vi "ferro fit.vi"(7 "ferro response parameters":T1 {"time const b (uS)" scale=0.0..200.0; "amplitude b (V)" scale=0.0..50.0; "time const a (uS)" scale=0.0..200.0; "amplitude a (V)" scale=0.0..50.0}, 11 "time array in (uS)":dbl[](array[numeric])) -> (0 "parameters array out":dbl[](array[numeric]), 2 "voltage array out (V)":dbl[](array[numeric]), 3 "time array out (uS)":dbl[](array[numeric]))   [LabVIEW 2017]
uses:
  typedefs/ferro response parameter cluster.ctl
panel:
  # "needs work\nsee BD"
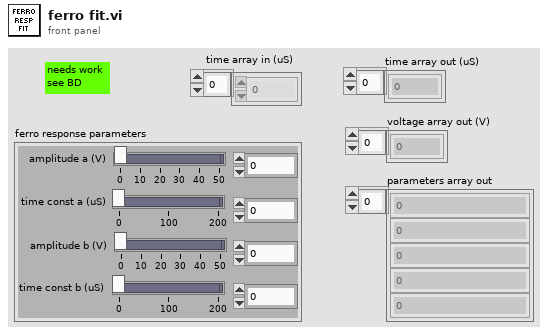
[diagram p1: front panel]
types:
  T1 = typedef "ferro response parameter cluster.ctl" = cluster{"amplitude a (V)":dbl, "time const a (uS)":dbl, "amplitude b (V)":dbl, "time const b (uS)":dbl}
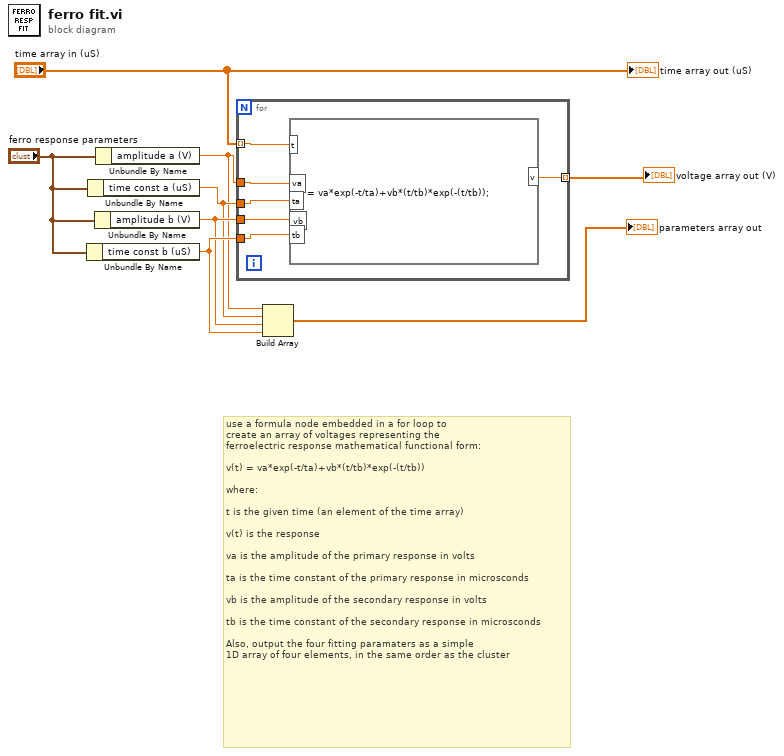
[diagram p0: block diagram]
diagram:
  # "use a formula node embedded in a for loop to \ncreate an array of voltages representing the \nferroelectric response mathematical functional form:\n\nv(t) = va*exp(-t/ta)+vb*(t/tb)*exp(-(t/tb))\n\nwhere:\n\nt is the given time (an element of the time array)\n\nv(t) is the response\n\nva is the amplitude of the primary response in volts\n\nta is the time constant of the primary response in microsconds\n\nvb is the amplitude of the secondary response in volts\n\ntb is the time constant of the secondary response in microsconds\n\nAlso, output the four fitting paramaters as a simple \n1D array of four elements, in the same order as the cluster"
  n1 = Unbundle By Name("ferro response parameters") -> ("time const b (uS)"=w6:dbl)
  n2 = Unbundle By Name("ferro response parameters") -> ("time const a (uS)"=w4:dbl)
  n3 = Unbundle By Name("ferro response parameters") -> ("amplitude b (V)"=w5:dbl)
  n4 = Unbundle By Name("ferro response parameters") -> ("amplitude a (V)"=w3:dbl)
  n5 = for {
    tunnel: w6 -> [w14]
    tunnel: w5 -> [w13]
    tunnel: w4 -> [w12]
    tunnel: w3 -> [w11]
    tunnel: "time array in (uS)" -> [w10] mode=indexing
    tunnel: [w9] -> w1 mode=indexing
    n6 = formula code="v = va*exp(-t/ta)+vb*(t/tb)*exp(-(t/tb));"("va"=w11, "ta"=w12, "vb"=w13, "tb"=w14, "t"=w10) -> ("v"=w9:dbl)
  }
  "voltage array out (V)" <- w1
  n7 = Build Array(w3, w4, w5, w6) -> (→"parameters array out":dbl[])
  "time array out (uS)" <- "time array in (uS)"
